vi "Get language tag.vi"() -> (3 "language tag":string)   [LabVIEW 2025, in "Full User Interface.lvlib"]
uses:
  Full User Interface.lvlib
  Key.ctl
  Localization/Localization.lvlib
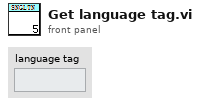
[diagram p1: front panel]
types:
  T1 = typedef "Full User Interface.lvlib/Key.ctl" = enum16{"Language", "Model"}
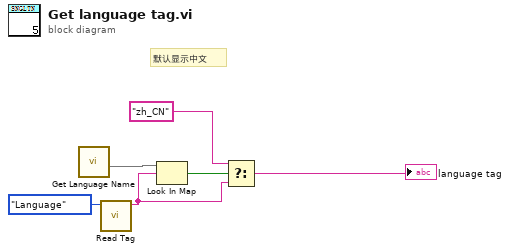
[diagram p0: block diagram]
diagram:
  # "默认显示中文"
  n1 = call "Get Language Name.vi"() -> ("Path"=w5:map{string, path})  [unwired: 8 in, 3 out]
  n2 = call "Read Tag.vi"("Enum"=Key."Language") -> ("value"=w3:string)  [unwired: 9 in, 1 out]
  n3 = Look In Map(map=w5, key=w3) -> (key not found?=w4:bool)  [unwired: 1 in, 1 out]
  n4 = Select(t="zh_CN" ("Language in"), s=w4, f=w3) -> (s? t:f=→"language tag":string)
